vi "Grid Map to Bool Array Test.vi"() -> ()   [LabVIEW 2017]
uses:
  Classes/ElectrodeGrid.lvclass
  Classes/ElectrodeGrid.lvclass/ElectrodeGrid.ctl
panel:
  out "Array":bool[](array[boolean])
  in  "stop":bool
  in  "SM Electrode Grid":bool[][](array[boolean])=[[FALSE, FALSE, FALSE, FALSE, FALSE, FALSE], [FALSE, FALSE, FALSE, FALSE, FALSE, FALSE], [FALSE, FALSE, FALSE, FALSE, FALSE, FALSE], [FALSE, FALSE, FALSE, FALSE, FALSE, FALSE], [FALSE, FALSE, FALSE, FALSE, FALSE, FALSE], [FALSE, FALSE, FALSE, FALSE, FALSE, FALSE]]
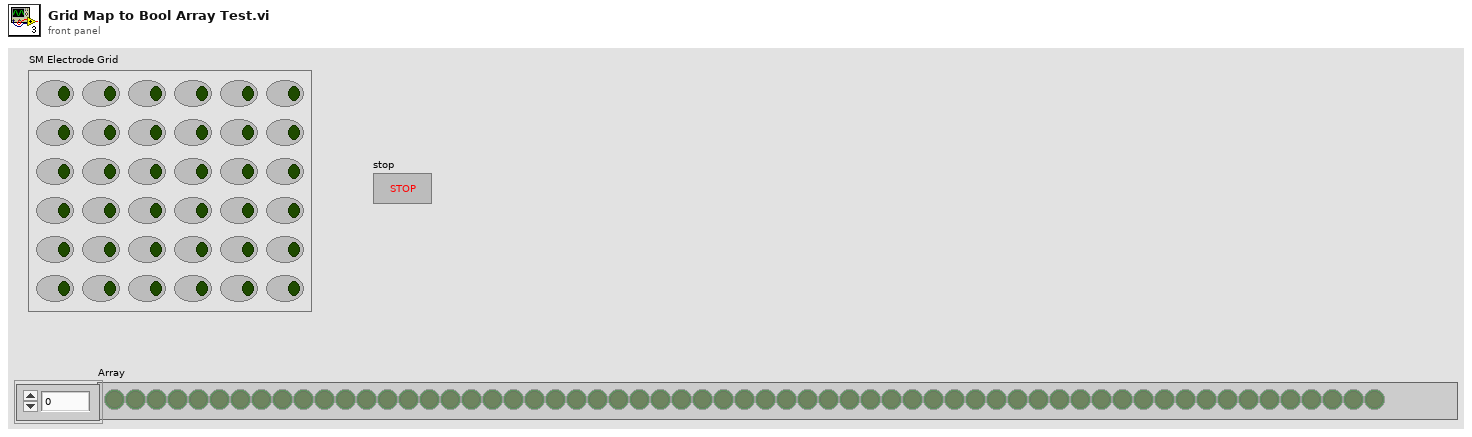
[diagram p1: front panel]
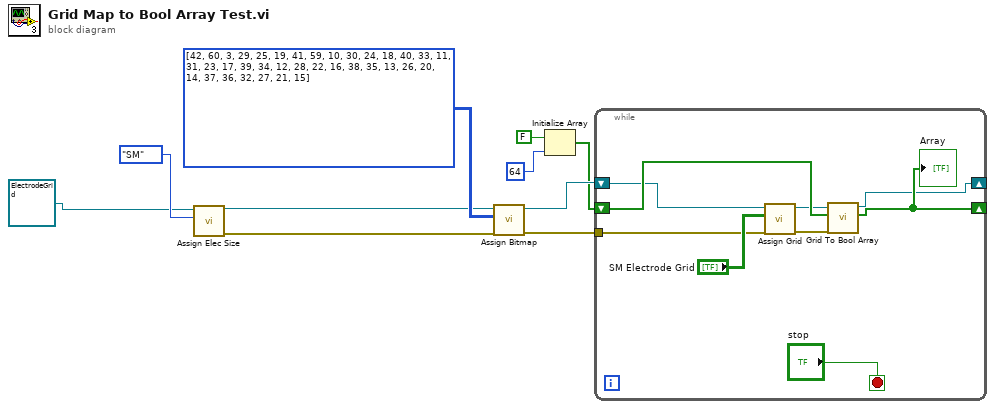
[diagram p0: block diagram]
diagram:
  n1 = call "Assign Elec Size.vi"("electrode size"=enum16{"XS", "SM", "LG"}."SM", "ElectrodeGrid in"=refnum<class "ElectrodeGrid.lvclass"> refnum ("ElectrodeGrid.lvclass")) -> ("error out"=w5:errorcluster, "ElectrodeGrid out"=w4:refnum<class "ElectrodeGrid.lvclass">)  [unwired: 8 in]
  n2 = call "Assign Bitmap.vi"("error in (no error)"=w5, "bitmap"=u8[][] [[42, 60, 3, 29, 25, 19], [41, 59, 10, 30, 24, 18], [40, 33, 11, 31, 23, 17], [39, 34, 12, 28, 22, 16], [38, 35, 13, 26, 20, 14], [37, 36, 32, 27, 21, 15]], "ElectrodeGrid in"=w4) -> ("error out"=w7:errorcluster, "ElectrodeGrid out"=w6:refnum<class "ElectrodeGrid.lvclass">)  [unwired: 7 in]
  n3 = Initialize Array(FALSE, 64 ("dimension size")) -> (w1:bool[])
  n4 = while {
    tunnel: w7 -> [w13]
    shift-right: [w12] -> _
    shift-left: w1 -> [w18]
    shift-right: [w11] -> _
    shift-left: w6 -> [w14]
    stop <- "stop" stop-if-true
    n5 = call "Assign Grid.vi"("error in (no error)"=w13, "grid"="SM Electrode Grid", "ElectrodeGrid in"=w14) -> ("error out"=w16:errorcluster, "ElectrodeGrid out"=w15:refnum<class "ElectrodeGrid.lvclass">)  [unwired: 7 in]
    n6 = call "Grid To Bool Array.vi"("error in (no error)"=w16, "Bool Array In"=w18, "ElectrodeGrid in"=w15) -> ("Bool Array Out"=w12:bool[], "ElectrodeGrid out"=w11:refnum<class "ElectrodeGrid.lvclass">)  [unwired: 6 in, 1 out]
    "Array" <- w12
  }
